vi "Init.vi"(8 "error in (no error)":errorcluster, 10 "Params":variant, 11 "PI650 VoltageAmp in":refnum<class "PI650 VoltageAmp.lvclass">) -> (0 "error out":errorcluster, 3 "PI650 VoltageAmp out":refnum<class "PI650 VoltageAmp.lvclass">)   [LabVIEW 2020, in "Pickering.lvlib" / "PI650 VoltageAmp.lvclass"]
uses:
  PI650 VoltageAmp.lvclass
  PI650 VoltageAmp.lvclass/PI650 VoltageAmp.ctl
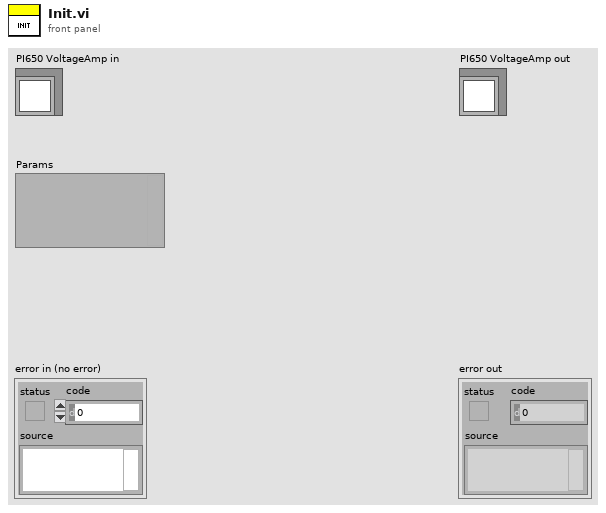
[diagram p1: front panel]
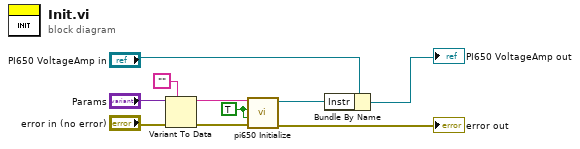
[diagram p0: block diagram]
diagram:
  w9 = TRUE ("reset device")
  n1 = Variant To Data(error in="error in (no error)", type="", Variant="Params") -> (data=w6:string, error out=w8:errorcluster)
  n2 = call <instrlib>:"pi650 Initialize.vi"("error in (no error)"=w8, "reset device (Reset Device)"=w9, "id query (Do Query)"=w9, "resource name"=w6) -> ("error out"=→"error out":errorcluster, "instrument handle out"=w10:refnum<visa-resource-name>)  [unwired: 6 in]
  n3 = Bundle By Name(cluster="PI650 VoltageAmp in", "Instr"=w10) -> (→"PI650 VoltageAmp out":refnum<class "PI650 VoltageAmp.lvclass">)
